vi "DLIWebPowerSwitch.vi"(4 "Scan Period":dbl format="%.2f", 5 "Previous Scan Value":dbl format="%.2f", 6 "Present scan array":dbl[](array[numeric]) format="%.2f", 7 "Value to Output":dbl format="%.2f", 8 "Ch Description":T1={"Ch Name"="Valve8", "Type"="DLI WebPowerSwitch", "Function"=enum."Relay Output", "Ch State"=enum."On", "Calibration type"="", "A"=200.0, "B"=0.0, "C"=0.0, "D"=0.0, "Comments"="", "Address"={"Main"=0, "Ch."=1, "Sub"=0, "Port Name"="192.168.126.155"}, "String"="LV:LV", "Duty"=65535} {"Duty" format="%016b"; "D" format="%#_5g"; "C" format="%#_5g"; "B" format="%#_5g"; "A" format="%#_5g"}, 9 "Ch names":string[](array[string])) -> (0 "Scan comment":string, 1 "Output":dbl format="%.3f", 3 "HelpText":string="Value to Output: 1-On 0-Off 99-Toggle\nOutput state is read back, and will be 0 for Off, 1 for On\n\"Port Name\" contains the IP address of the unit\nCh. is used to specify the outlet number, 1-8\nComment (the red box) is used for username:password\n\"A\" is the timeout, in ms")   [LabVIEW 2016]
uses:
  ADAM Client/Sub VIs/ADAM Controls/Ch_description_ADAM.ctl
  ADAM Client/Sub VIs/ADAM Controls/Module_type_ADAM.ctl
  ADAM Client/Sub VIs/ADAM Controls/Function_ADAM.ctl
  ADAM Client/Sub VIs/ADAM Controls/Channel_State.ctl
  ADAM Client/Sub VIs/ADAM Controls/Calib_type_ADAM.ctl
  ADAM Client/Sub VIs/ADAM Controls/Address.ctl
  <vilib>/Utility/error.llb/DialogType.ctl
  <vilib>/httpClient/LabVIEWHTTPClient.lvlib
panel:
  out "body":string
  out "headers":string
  # "VI to control the Digital Loggers International Web Power Switch"
  # "https://www.digital-loggers.com/lpc.html"
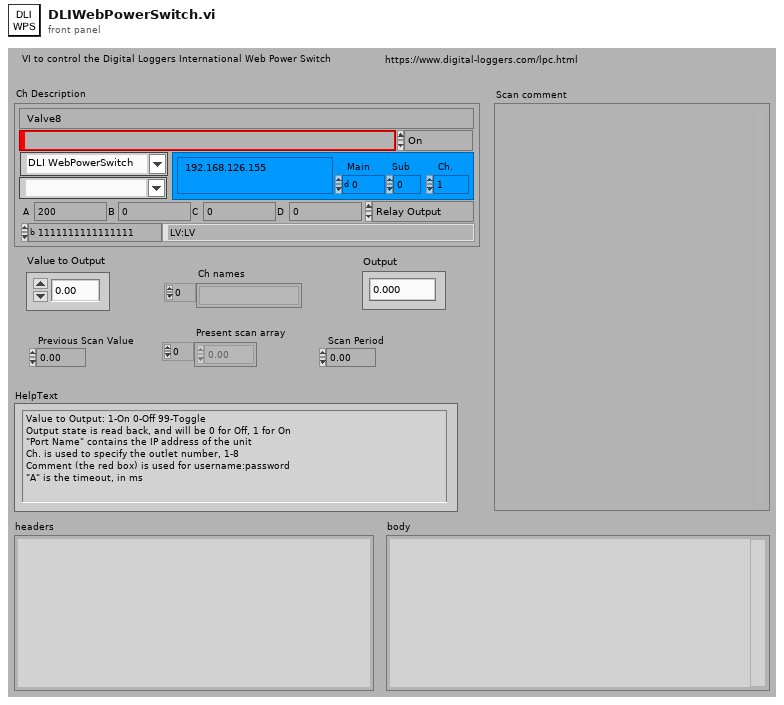
[diagram p1: front panel]
types:
  T1 = typedef "Ch_description_ADAM.ctl" = cluster{"Ch Name":string, "Type":T2, "Function":T3, "Ch State":T4, "Calibration type":T5, "A":dbl, "B":dbl, "C":dbl, "D":dbl, "Comments":string, "Address":T6, "String":string, "Duty":u16}
  T2 = typedef "Module_type_ADAM.ctl" = string
  T3 = typedef "Function_ADAM.ctl" = enum16{"Analogue Input", "Digital Input", "Event counter", "Event rate", "Analogue Output", "Digital Output", "Relay Output"}
  T4 = typedef "Channel_State.ctl" = enum16{"On", "Off", "Always On", "Always Off"}
  T5 = typedef "Calib_type_ADAM.ctl" = string
  T6 = typedef "Address.ctl" = cluster{"Main":i32, "Ch.":i32, "Sub":i32, "Port Name":string}
  T7 = typedef "DialogType.ctl" = u16
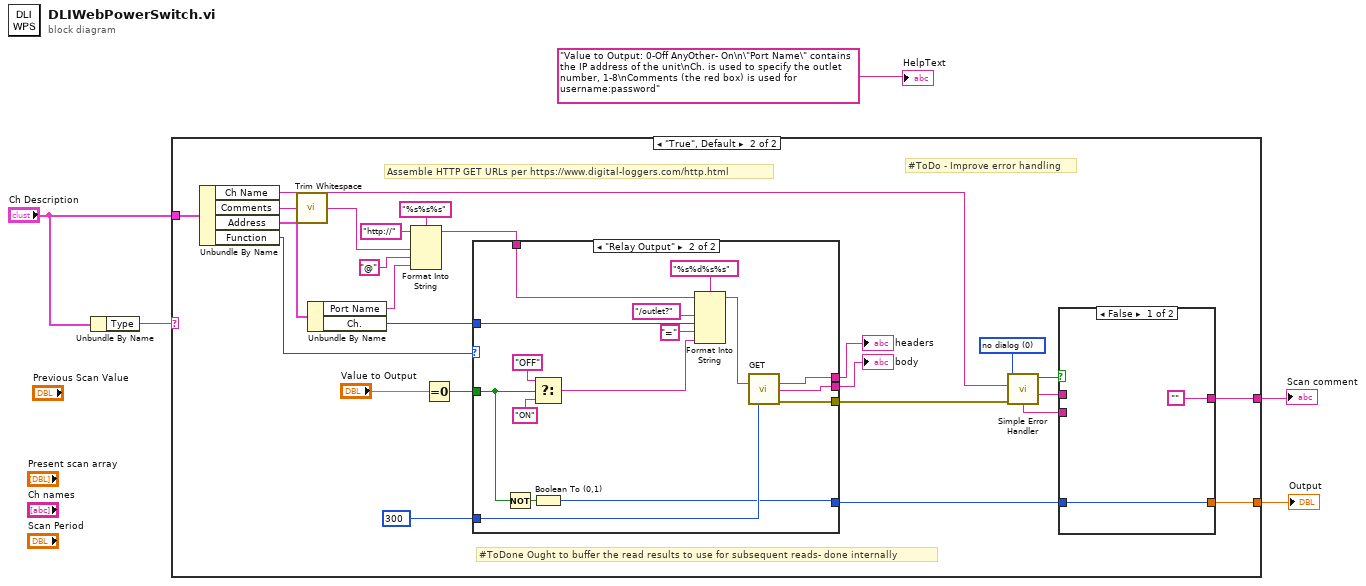
[diagram p0: block diagram]
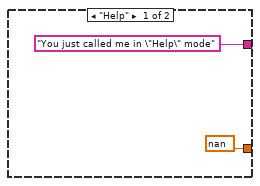
[diagram p2: hidden frame]
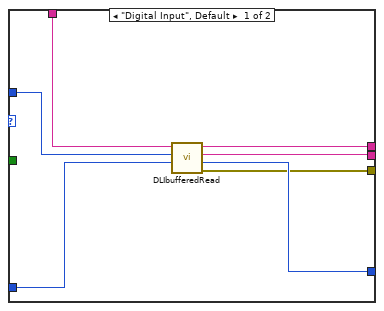
[diagram p3: hidden frame]
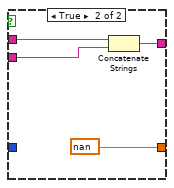
[diagram p4: hidden frame]
diagram:
  n1 = Unbundle By Name("Ch Description") -> ("Type"=w2:T2)
  n2 = case shown="\"True\", Default" w2 {
    tunnel: ["You just called me in \"Help\" mode" w27] -> w5
    tunnel: [nan ("t") w26] -> w4
    tunnel: "Ch Description" -> [_ w18]
    frame "Help" {
    }
    frame "True", Default {
      w32 = T7 0 items=["no dialog", "OK message", "continue or stop message", "OK message + warnings", "continue/stop + warnings"] ("type of dialog (OK msg:1)")
      # "#ToDone Ought to buffer the read results to use for subsequent reads- done internally"
      # "#ToDo - Improve error handling"
      # "Assemble HTTP GET URLs per https://www.digital-loggers.com/http.html"
      n3 = Unbundle By Name(w18) -> ("Ch Name"=w19:string, "Comments"=w12:string, "Address"=w29:T6, "Function"=w15:T3)
      n4 = call <vilib>:"Trim Whitespace.vi"("string"=w12) -> ("trimmed string"=w11:string)  [unwired: 1 in]
      n5 = Unbundle By Name(w29) -> ("Port Name"=w23:string, "Ch."=w20:i32)
      n6 = Format Into String(format string="%s%s%s", initial string="http://", w11, "@" ("input 2"), w23) -> (resulting string=w21:string)  [unwired: 1 in, 1 out]
      n7 = Equal To 0?(x="Value to Output") -> (x = 0?=w9:bool)
      n8 = case shown="\"Relay Output\"" w15 {
        tunnel: [w33 w51] -> w14
        tunnel: w21 -> [w39 w50]
        tunnel: w20 -> [w38 w49]
        tunnel: 300 ("A") -> [w37 w46]
        tunnel: [w36 w48] -> w17
        tunnel: [w35 w47] -> w16
        tunnel: [w34 w41] -> w13
        tunnel: w9 -> [_ w42]
        frame "Digital Input", Default {
          n9 = call "DLIbufferedRead.vi"("timeout(ms)"=w37, "Ch."=w38, "URL"=w39) -> ("error out"=w33:errorcluster, "state(1or0)"=w34:i16, "body"=w35:string, "headers"=w36:string)  [unwired: 5 in]
        }
        frame "Relay Output" {
          n10 = Not(x=w42) -> (.not. x?=w40:bool)
          n11 = Select(t="OFF", s=w42, f="ON") -> (s? t:f=w43:string)
          n12 = Boolean To (0,1)(Boolean=w40) -> (0, 1=w41:i16)
          n13 = Format Into String(format string="%s%d%s%s", initial string=w50, "/outlet?" ("input 4"), w49, "=", w43) -> (resulting string=w52:string)  [unwired: 1 in, 1 out]
          n14 = call <vilib>:"GET.vi"("url"=w52, "timeout (10000)"=w46) -> ("headers"=w48:string, "body"=w47:string, "error out"=w51:errorcluster)  [unwired: 10 in, 1 out]
        }
      }
      "headers" <- w17
      "body" <- w16
      n15 = call <vilib>:"Simple Error Handler.vi"("error source (\" \")"=w19, "type of dialog (OK msg:1)"=w32, "error in (no error)"=w14) -> ("error?"=w28:bool, "source out"=w30:string, "message"=w31:string)  [unwired: 4 out]
      n16 = case shown="False" w28 {
        tunnel: w31 -> [_ w59]
        tunnel: w30 -> [_ w60]
        tunnel: ["" w58] -> w27
        tunnel: [w56 nan ("t")] -> w26
        tunnel: w13 -> [w56 _]
        frame False {
        }
        frame True {
          n17 = Concatenate Strings(w60, w59) -> (w58:string)
        }
      }
    }
  }
  "Output" <- w4
  "Scan comment" <- w5
  "HelpText" <- "Value to Output: 0-Off AnyOther- On\n\"Port Name\" contains the IP address of the unit\nCh. is used to specify the outlet number, 1-8\nComments (the red box) is used for username:password"
